vi "sonde front panel_1.vi"() -> ()   [LabVIEW 2015]
panel:
  in  "Write Data to Spreadsheet":bool
  out "ORP":dbl
  out "pH":dbl
  out "Dissolved\nOxygen":dbl
  out "Specific\nConductance":dbl
  out "Cumulative\nVolume":dbl
  in  "Sample Not Collected":bool
  in  "Record Values":bool
  in  "Tab Control":T1(tab)
  out "Temporary Data Files Directory 2":path
  in  "Data File Directory":path
  out "Array":string[][](array[string])
  in  "Write Data to Spreadsheet 2":bool
  in  "Select Reasons to Record Data":u16(ring) items=["Per Client Request", "Timed Out", "Sample stopped flowing", "Equipment Issue"]
  out "Current Time (s)":dbl
  out "Current Depth (ft)":dbl
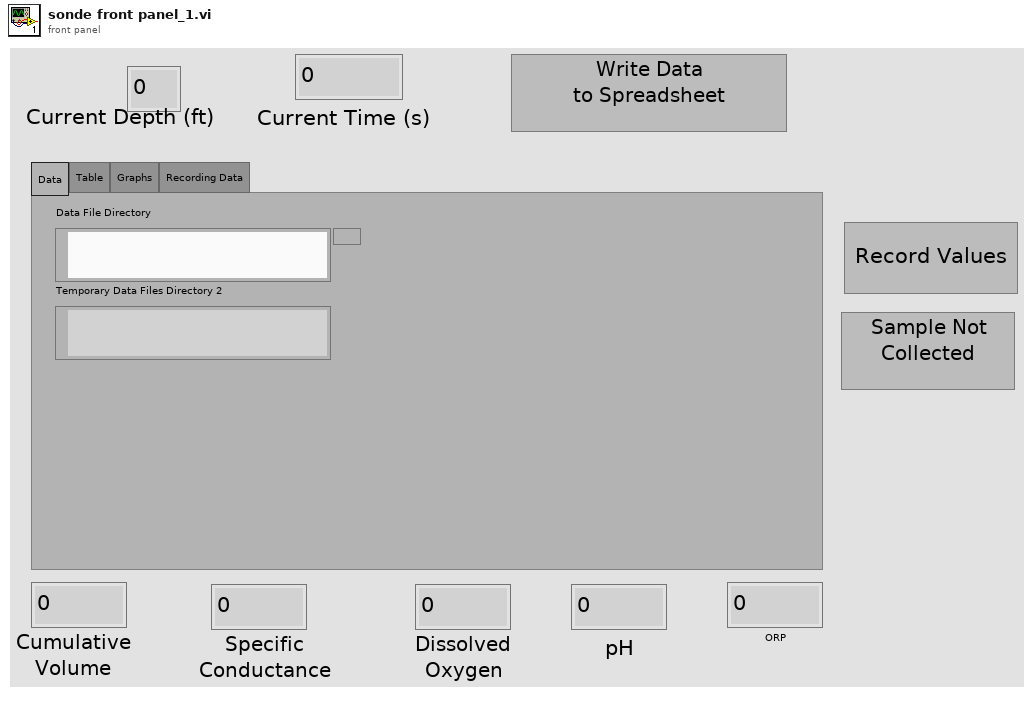
[diagram p1: front panel]
types:
  T1 = enum32{"Data", "Table", "Graphs", "Recording Data"}
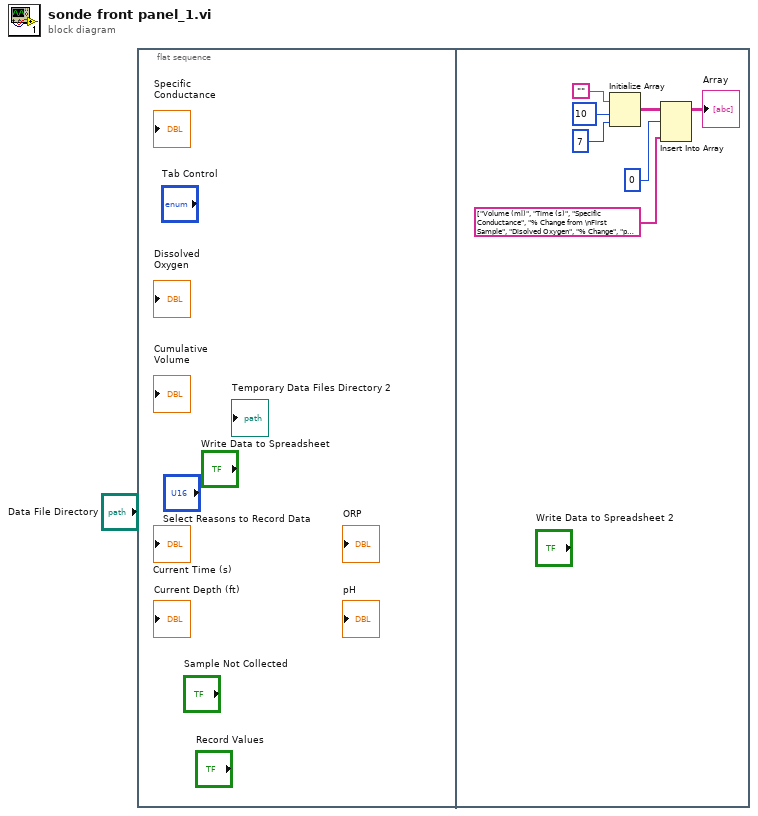
[diagram p0: block diagram]
diagram:
  n1 = flat-sequence {
    frame #0 {
    }
    frame #1 {
      n2 = Initialize Array("", 10 ("dimension size"), 7 ("dimension size")) -> (w2:string[][])
      n3 = Insert Into Array(array=w2, index (row)=0, new element=string[] ["Volume (ml)", "Time (s)", "Specific Conductance", "% Change from \nFirst Sample", "Disolved Oxygen", "% Change", "pH", "% Change", "ORP", "% Change"]) -> (→"Array":string[][])  [unwired: 1 in]
    }
  }
